vi "Simulate Angular Position.vi"() -> (1 "Present (s)":dbl, 2 "Gauge":dbl(knob) scale=-180.0..180.0)   [LabVIEW 2019]
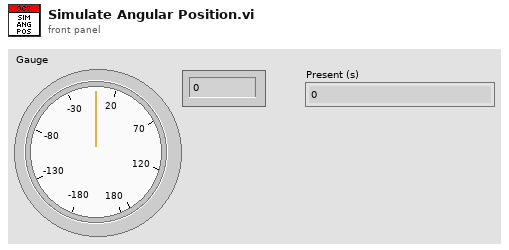
[diagram p1: front panel]
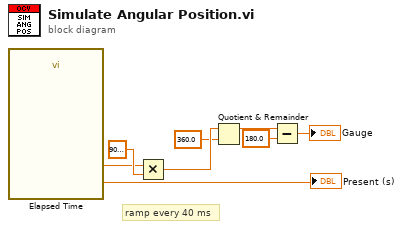
[diagram p0: block diagram]
diagram:
  # "ramp every 40 ms"
  n1 = call "Elapsed Time"() -> ("Present (s)"=→"Present (s)":dbl, "Elapsed Time (s)"=w1:dbl)  [unwired: 12 in, 6 out]
  n2 = Multiply(x=w1, y=9000.0) -> (x*y=w3:dbl)
  n3 = Quotient & Remainder(x=w3, y=360.0) -> (x-y*floor(x/y)=w4:dbl)  [unwired: 1 out]
  n4 = Subtract(x=w4, y=180.0) -> (x-y=→"Gauge":dbl)
